vi "Search for Deepest Nested Parenthesis Pairs.vi"(8 "Error In":errorcluster, 9 "offset":i32, 11 "Formula String":string) -> (0 "Error Out":errorcluster, 1 "Array of Parenthesis Pairs":cluster{"Start Index":i32, "Stop Index":i32}[](array[cluster]), 2 "Unmatched Open Parenthesis?":bool, 3 "Formula String (dup)":string, 5 "Unmatched Close Parenthesis?":bool)   [LabVIEW 2021, in "Formula.lvlib"]
uses:
  Formula.lvlib
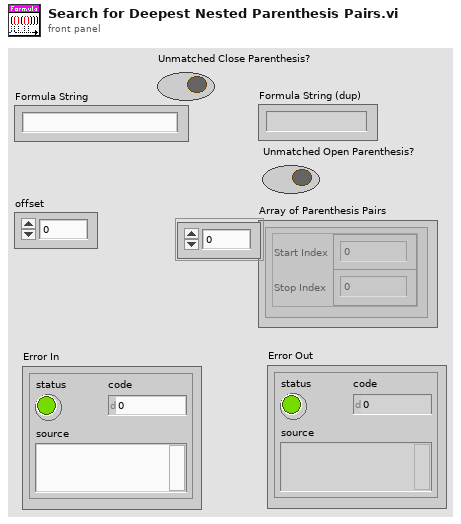
[diagram p1: front panel]
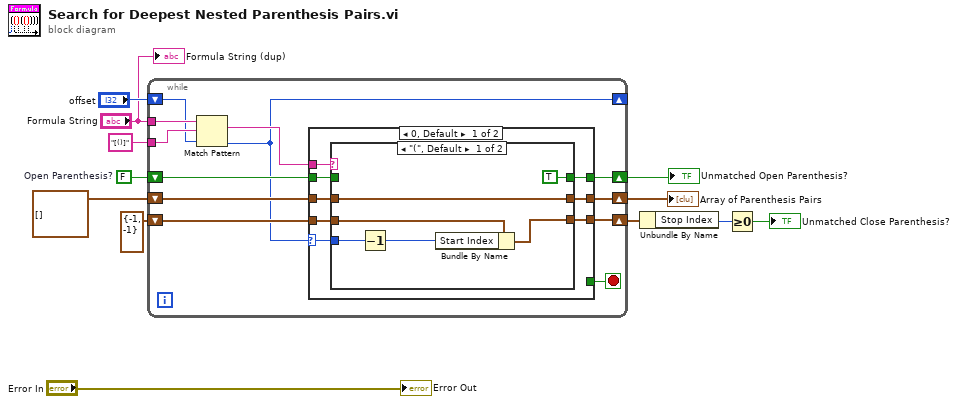
[diagram p0: block diagram]
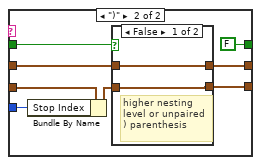
[diagram p2: hidden frame]
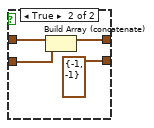
[diagram p3: hidden frame]
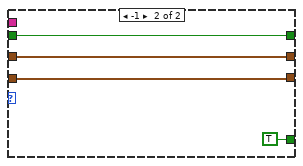
[diagram p4: hidden frame]
diagram:
  w9 = FALSE  # Open Parenthesis?
  n1 = while {
    shift-right: [w13] -> _
    shift-left: "offset" -> [w14]
    shift-right: [w15] -> w7
    shift-left: cluster{"Start Index":i32, "Stop Index":i32}[] [] ("Array of Parenthesis Pair") -> [w16]
    tunnel: "[()]" ("regular expression") -> [w22]
    shift-right: [w19] -> w4
    shift-left: w9 -> [w20]
    shift-right: [w17] -> w3
    shift-left: cluster{"Start Index":i32, "Stop Index":i32} {"Start Index"=-1, "Stop Index"=-1} ("Parenthesis Pair Indices") -> [w18]
    tunnel: "Formula String" -> [w23]
    stop <- w24 stop-if-true
    n2 = Match Pattern(string=w23, regular expression=w22, offset (0)=w14) -> (match substring=w21:string, offset past match=w13:i32)  [unwired: 2 out]
    n3 = case shown="0, Default" w13 {
      selector: w13 -> [w25 _]
      tunnel: [_ TRUE] -> w24
      tunnel: w21 -> [w32 _]
      tunnel: w20 -> [w31 w55]
      tunnel: [w30 w55] -> w19
      tunnel: w18 -> [w29 w53]
      tunnel: [w28 w53] -> w17
      tunnel: w16 -> [w27 w54]
      tunnel: [w26 w54] -> w15
      frame 0, Default {
        n4 = case shown="\"(\", Default" w32 {
          tunnel: w25 -> [w37 w46]
          tunnel: w31 -> [_ w41]
          tunnel: [TRUE ("Open Parenthesis?") FALSE ("Open Parenthesis?")] -> w30
          tunnel: w29 -> [w36 w45]
          tunnel: [w35 w39] -> w28
          tunnel: w27 -> [w34 w44]
          tunnel: [w34 w43] -> w26
          frame "(", Default {
            n5 = Decrement(x=w37) -> (x-1=w33:i32)
            n6 = Bundle By Name(cluster=w36, "Start Index"=w33) -> (w35:cluster{"Start Index":i32, "Stop Index":i32})
          }
          frame ")" {
            n7 = Bundle By Name(cluster=w45, "Stop Index"=w46) -> (w42:cluster{"Start Index":i32, "Stop Index":i32})
            n8 = case shown="False" w41 {
              tunnel: w44 -> [w48 w52]
              tunnel: [w48 w51] -> w43
              tunnel: w42 -> [w47 w50]
              tunnel: [w47 cluster{"Start Index":i32, "Stop Index":i32} {"Start Index"=-1, "Stop Index"=-1} ("Parenthesis Pair Indices")] -> w39
              frame False {
                # "higher nesting\nlevel or unpaired\n) parenthesis"
              }
              frame True {
                n9 = Build Array (concatenate)(w52, w50) -> (w51:cluster{"Start Index":i32, "Stop Index":i32}[])
              }
            }
          }
        }
      }
      frame -1 {
      }
    }
  }
  "Array of Parenthesis Pairs" <- w7
  "Unmatched Open Parenthesis?" <- w4
  n10 = Unbundle By Name(w3) -> ("Stop Index"=w2:i32)
  n11 = Greater Or Equal To 0?(x=w2) -> (x >= 0?=→"Unmatched Close Parenthesis?":bool)
  "Formula String (dup)" <- "Formula String"
  "Error Out" <- "Error In"
